vi "LJM logger errors to message.vi"(2 "Scaling Error":errorcluster, 3 "LJM Error":errorcluster) -> (0 "Error Message":string="No Error", 1 "status":bool)   [LabVIEW 2026]
uses:
  <vilib>/Utility/error.llb/DialogType.ctl
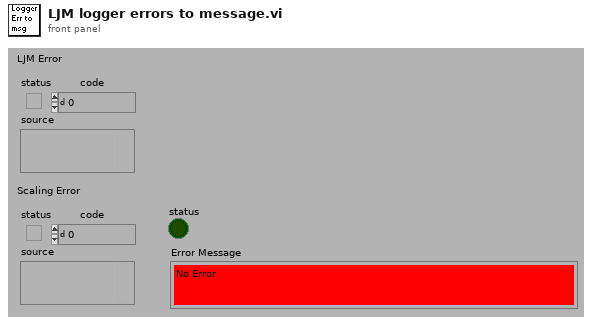
[diagram p1: front panel]
types:
  T1 = typedef "DialogType.ctl" = u16
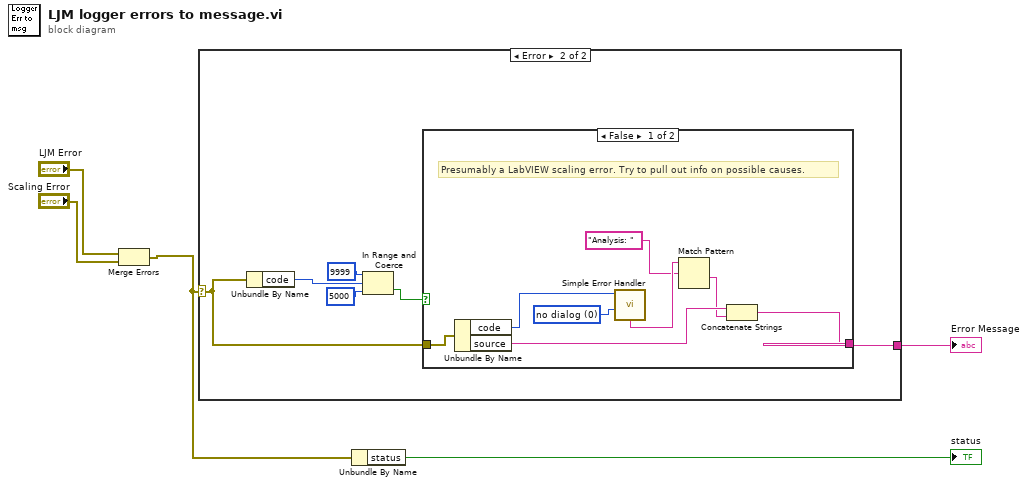
[diagram p0: block diagram]
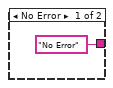
[diagram p2: hidden frame]
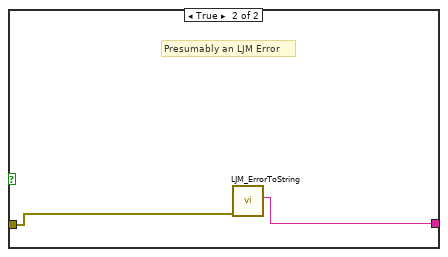
[diagram p3: hidden frame]
diagram:
  n1 = Merge Errors("LJM Error", "Scaling Error") -> (w1:errorcluster)
  n2 = case shown="Error" w1 {
    selector: w1 -> [_ w7]
    tunnel: ["No Error" ("String") w8] -> w3
    frame No Error {
    }
    frame Error {
      n3 = Unbundle By Name(w7) -> ("code"=w10:i32)
      n4 = In Range and Coerce(upper limit=9999, x=w10, lower limit=5000) -> (In Range?=w9:bool)  [unwired: 1 out]
      n5 = case shown="False" w9 {
        tunnel: [w19 w21] -> w8
        tunnel: w7 -> [w18 w22]
        frame False {
          w14 = T1 0 items=["no dialog", "OK message", "continue or stop message", "OK message + warnings", "continue/stop + warnings"] ("type of dialog (OK msg:1)")
          # "Presumably a LabVIEW scaling error. Try to pull out info on possible causes."
          n6 = Unbundle By Name(w18) -> ("code"=w15:i32, "source"=w20:string)
          n7 = call <vilib>:"Simple Error Handler.vi"("error code (no error:0)"=w15, "type of dialog (OK msg:1)"=w14) -> ("message"=w17:string)  [unwired: 3 in, 4 out]
          n8 = Match Pattern(string=w17, regular expression="Analysis: ") -> (after substring=w13:string)  [unwired: 1 in, 3 out]
          n9 = Concatenate Strings(w20, w13) -> (w19:string)
        }
        frame True {
          # "Presumably an LJM Error"
          n10 = call "LJM_ErrorToString.vi"("error in"=w22) -> ("String"=w21:string)  [unwired: 10 in]
        }
      }
    }
  }
  "Error Message" <- w3
  n11 = Unbundle By Name(w1) -> ("status"=→"status":bool)
